vi "PH_Revolver-GUI_6P.set Revolver Position.vi"(0 "VI in":refnum<vi>, 2 "Revolver Position":T1 items=["unknown", "Position 0", "Position 60", "Position 120", "Position 180", "Position 240", "Position 300", "moving"], 5 "error in (no error)":errorcluster) -> (14 "VI out":refnum<vi>, 19 "error out":errorcluster)   [LabVIEW 2014, in "PH_Revolver-GUI_6P.lvlib"]
uses:
  PH_Revolver-GUI_6P.lvlib
  PH_Revolver-GUI_6P.Position.ctl
  CSlibraries-extern/DimLVEvent/LVDimInterface/LVDimInterface.lvlib
  PH_Basics/PH_Common/PH_Common.lvlib
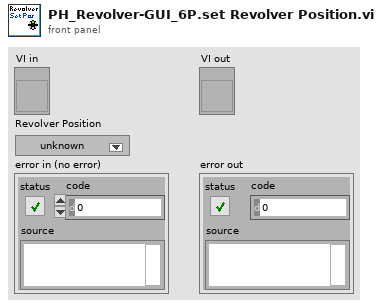
[diagram p1: front panel]
types:
  T1 = typedef "PH_Revolver-GUI_6P.lvlib/PH_Revolver-GUI_6P.Position.ctl" = u16
  T2 = typedef "PH_Revolver-GUI_6P.lvlib/PH_Revolver-GUI_6P.i attribute.ctl" = cluster{"GUI Refs":cluster{"0°":refnum<vi>, "60°":refnum<vi>, "120°":refnum<vi>, "180°":refnum<vi>, "240°":refnum<vi>, "300°":refnum<vi>, "Action":refnum<vi>}, "Revolver Position":T1, "Service ID Position":i32, "Captions":string[]}
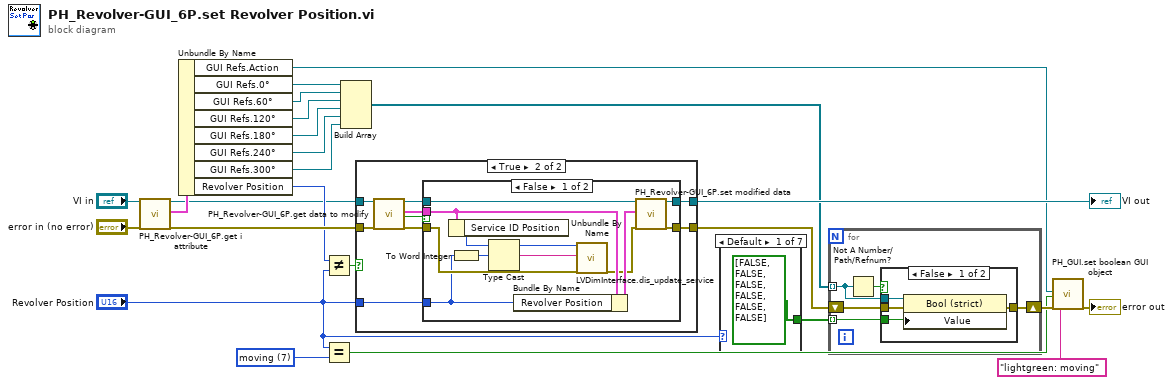
[diagram p0: block diagram]
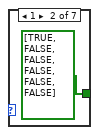
[diagram p2: hidden frame]
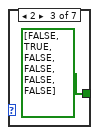
[diagram p3: hidden frame]
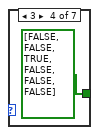
[diagram p4: hidden frame]
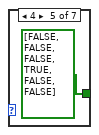
[diagram p5: hidden frame]
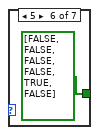
[diagram p6: hidden frame]
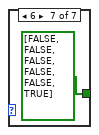
[diagram p7: hidden frame]
diagram:
  w6 = T1 7 items=["unknown", "Position 0", "Position 60", "Position 120", "Position 180", "Position 240", "Position 300", "moving"] ("Revolver Position")
  n1 = call "PH_Revolver-GUI_6P.get i attribute.vi"("i ref in"="VI in", "error in (no error)"="error in (no error)") -> ("i ref out"=w18:refnum<vi>, "i attribute"=w21:T2, "error out"=w23:errorcluster)  [unwired: 15 in]
  n2 = Unbundle By Name(w21) -> ("GUI Refs.Action"=w3:refnum<vi>, "GUI Refs.0°"=w16:refnum<vi>, "GUI Refs.60°"=w15:refnum<vi>, "GUI Refs.120°"=w14:refnum<vi>, "GUI Refs.180°"=w13:refnum<vi>, "GUI Refs.240°"=w12:refnum<vi>, "GUI Refs.300°"=w11:refnum<vi>, "Revolver Position"=w20:T1)
  n3 = Not Equal?(x=w20, y="Revolver Position") -> (x != y?=w17:bool)
  n4 = Equal?(x="Revolver Position", y=w6) -> (x = y?=w2:bool)
  n5 = Build Array(w16, w15, w14, w13, w12, w11) -> (w8:refnum<vi>[])
  n6 = case shown="True" w17 {
    tunnel: w23 -> [w25 w35]
    tunnel: [w26 w34] -> w19
    tunnel: w18 -> [w26 w33]
    tunnel: [w25 w31] -> w7
    tunnel: "Revolver Position" -> [_ w28]
    frame False {
    }
    frame True {
      n7 = call "PH_Revolver-GUI_6P.get data to modify.vi"("i ref in"=w33, "error in (no error)"=w35) -> ("i ref out"=w32:refnum<vi>, "i attribute"=w30:T2, "timed out"=w27:bool, "error out"=w29:errorcluster)  [unwired: 14 in]
      n8 = case shown="False" w27 {
        tunnel: [w46 w48] -> w34
        tunnel: w32 -> [w45 w48]
        tunnel: [w44 w47] -> w31
        tunnel: w30 -> [w40 _]
        tunnel: w29 -> [w38 w47]
        tunnel: w28 -> [w36 _]
        frame False {
          n9 = Unbundle By Name(w40) -> ("Service ID Position"=w39:i32)
          n10 = To Word Integer(number=w36) -> (16bit integer=w41:i16)
          n11 = Type Cast(x=w41) -> (*(type *) &x=w42:string)  [unwired: 1 in]
          n12 = Bundle By Name(cluster=w40, "Revolver Position"=w36) -> (w43:T2)
          n13 = call "LVDimInterface.dis_update_service.vi"("my_serviceID"=w39, "data"=w42, "error in (no error)"=w38) -> ("error out"=w37:errorcluster)  [unwired: 14 in, 2 out]
          n14 = call "PH_Revolver-GUI_6P.set modified data.vi"("i ref in"=w45, "i attribute"=w43, "error in (no error)"=w37) -> ("i ref out"=w46:refnum<vi>, "error out"=w44:errorcluster)  [unwired: 15 in]
        }
        frame True {
        }
      }
    }
  }
  "VI out" <- w19
  n15 = case shown="Default" "Revolver Position" {
    tunnel: [bool[] [FALSE, FALSE, FALSE, FALSE, FALSE, FALSE] bool[] [TRUE, FALSE, FALSE, FALSE, FALSE, FALSE] bool[] [FALSE, TRUE, FALSE, FALSE, FALSE, FALSE] bool[] [FALSE, FALSE, TRUE, FALSE, FALSE, FALSE] bool[] [FALSE, FALSE, FALSE, TRUE, FALSE, FALSE] bool[] [FALSE, FALSE, FALSE, FALSE, TRUE, FALSE] bool[] [FALSE, FALSE, FALSE, FALSE, FALSE, TRUE]] -> w9
    frame Default {
    }
    frame 1 {
    }
    frame 2 {
    }
    frame 3 {
    }
    frame 4 {
    }
    frame 5 {
    }
    frame 6 {
    }
  }
  n16 = for {
    shift-right: [w59] -> w10
    shift-left: w7 -> [w60]
    tunnel: w8 -> [w57] mode=indexing
    tunnel: w9 -> [w56] mode=indexing
    n17 = Not A Number/Path/Refnum?(number/path/refnum=w57) -> (NaN/Path/Refnum?=w58:bool)
    n18 = case shown="False" w58 {
      tunnel: w60 -> [w64 w65]
      tunnel: [w63 w65] -> w59
      tunnel: w57 -> [w62 _]
      tunnel: w56 -> [w61 _]
      frame False {
        n19 = property class="Bool (strict)"(reference=w62, error in=w64, "Value"=w61) -> (error out=w63:errorcluster)  [unwired: 1 out]
      }
      frame True {
      }
    }
  }
  n20 = call "PH_GUI.set boolean GUI object.vi"("Boolean Knob GUI Ref"=w3, "Value"=w2, "error in (no error)"=w10, "Tip Strip"="lightgreen: moving") -> ("error out"=→"error out":errorcluster)  [unwired: 15 in]
